vi "Add Dependent File Property.vi"(6 "Node Type":string, 9 "Existing Property Names":string[](array[string]), 10 "Property Parent":string, 11 "Doc Ref":refnum<k20>) -> (1 "Cancelled?":bool, 3 "Property Name out":string, 4 "Node Found?":bool, 5 "Updated Node Ref":refnum<k20>)   [LabVIEW 2025]
panel:
  in  "RT Destination":string
  in  "SupportedTarget":string(combo)="All" caption="Supported Target"
  in  "Version":string
  in  "FIle Path":string
  in  "FileType":string(combo)="To Application Data Dir" caption="File Type"
  in  "ForceDownload":string(combo)="false" caption="Force Download"
  in  "Cancel Button":bool
  in  "Ok Button":bool
  in  "Documentation":string
  in  "Name":string
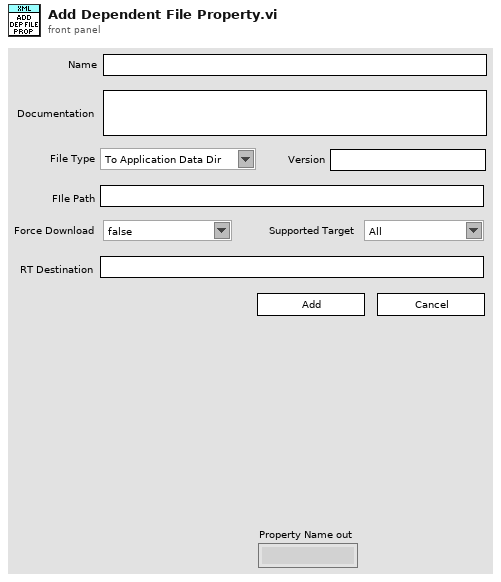
[diagram p1: front panel]
types:
  T1 = cluster{"Name":string, "Documentation":string, "FileType":string, "Version":string, "FIle Path":string, "ForceDownload":string, "SupportedTarget":string, "RT Destination":string}
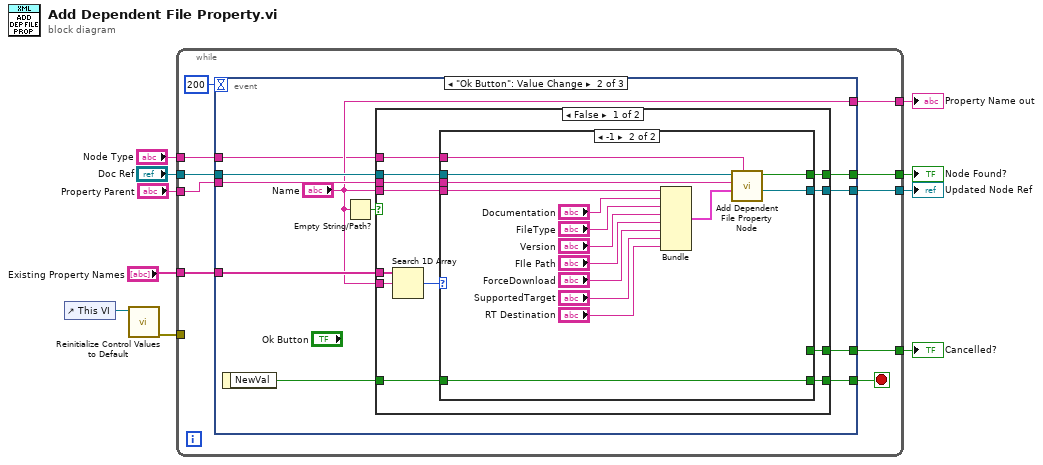
[diagram p0: block diagram]
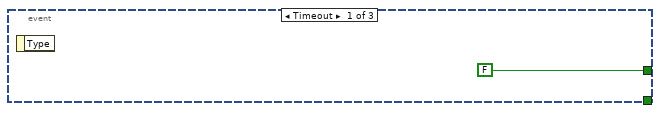
[diagram p2: hidden frame]
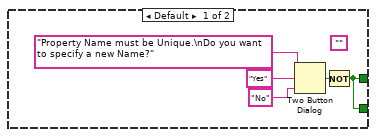
[diagram p3: hidden frame]
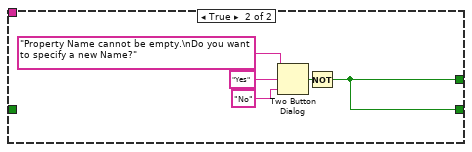
[diagram p4: hidden frame]
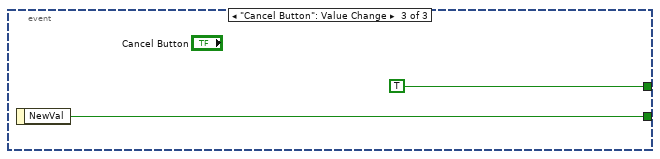
[diagram p5: hidden frame]
diagram:
  n1 = control-ref of="This VI"() -> (w9:refnum<vi>)
  n2 = call "Reinitialize Control Values to Default.vi"("VI Ref"=w9) -> ("error out"=w2:errorcluster)  [unwired: 10 in]
  n3 = while {
    tunnel: "Doc Ref" -> [w20]
    tunnel: [w18] -> w10
    tunnel: "Existing Property Names" -> [w16]
    tunnel: "Property Parent" -> [w15]
    tunnel: [w14] -> w6
    tunnel: [w13] -> w5
    tunnel: "Node Type" -> [w12]
    tunnel: w2 -> [_]
    tunnel: [w11] -> w1
    stop <- w17 stop-if-true
    n4 = event shown="[1] \"Ok Button\": Value Change" {
      selector: _ -> [_ _ _]
      dyn-events: _ -> [_ _ _]
      timeout: 200 -> [_ _ _]
      tunnel: [_ w28 w71] -> w17
      tunnel: w20 -> [_ w31 _]
      tunnel: [FALSE w30 TRUE] -> w18
      tunnel: w16 -> [_ w27 _]
      tunnel: w15 -> [_ w26 _]
      tunnel: [_ "Name" _] -> w14
      tunnel: [_ w24 _] -> w13
      tunnel: w12 -> [_ w23 _]
      tunnel: [_ w22 _] -> w11
      event Timeout {
        n5 = event-data() -> ()  [unwired: 1 in, 1 out]
      }
      event "Ok Button": Value Change {
        n6 = event-data() -> ("NewVal"=w29:bool)  [unwired: 1 in]
        n7 = Empty String/Path?(string/path="Name") -> (empty?=w32:bool)
        n8 = case shown="False" w32 {
          tunnel: w31 -> [w44 _]
          tunnel: "Name" -> [w38 _]
          tunnel: [w43 w65] -> w30
          tunnel: "Name" -> [w42 _]
          tunnel: w29 -> [w41 _]
          tunnel: [w40 w65] -> w28
          tunnel: w27 -> [w39 _]
          tunnel: w26 -> [w36 _]
          tunnel: [w35 _] -> w24
          tunnel: w23 -> [w34 _]
          tunnel: [w33 _] -> w22
          frame False {
            n9 = Search 1D Array(1D array=w39, element=w38) -> (index of element=w37:i32)  [unwired: 1 in]
            n10 = case shown="-1" w37 {
              tunnel: w44 -> [_ w63]
              tunnel: [w45 _] -> w43
              tunnel: w42 -> [_ w59]
              tunnel: [w45 w64] -> w40
              tunnel: w41 -> [_ w64]
              tunnel: w36 -> [_ w62]
              tunnel: [_ w61] -> w35
              tunnel: w34 -> [_ w60]
              tunnel: [_ w50] -> w33
              frame Default {
                (unwired) ""
                n11 = Two Button Dialog(message="Property Name must be Unique.\nDo you want to specify a new Name?" ("Errors"), 1:"No" ("F button name (\"Cancel\")"), 2:"Yes" ("T button name (\"OK\")")) -> (T button?=w46:bool)
                n12 = Not(x=w46) -> (.not. x?=w45:bool)
              }
              frame -1 {
                n13 = Bundle("Name"=w59, "Documentation"="Documentation", "FileType"="FileType", "Version"="Version", "FIle Path"="FIle Path", "ForceDownload"="ForceDownload", "SupportedTarget"="SupportedTarget", "RT Destination"="RT Destination") -> (w51:T1)  [unwired: 1 in]
                n14 = call "Add Dependent File Property Node.vi"("Node Type"=w60, "Dependent File Inputs"=w51, "Property Parent"=w62, "Doc Ref"=w63) -> ("Updated Node Ref"=w50:refnum<k20>, "Node Found?"=w61:bool)  [unwired: 6 in]
              }
            }
          }
          frame True {
            (unwired) ""
            n15 = Two Button Dialog(message="Property Name cannot be empty.\nDo you want to specify a new Name?" ("Errors"), 1:"No" ("F button name (\"Cancel\")"), 2:"Yes" ("T button name (\"OK\")")) -> (T button?=w67:bool)
            n16 = Not(x=w67) -> (.not. x?=w65:bool)
          }
        }
      }
      event "Cancel Button": Value Change {
        n17 = event-data() -> ("NewVal"=w71:bool)  [unwired: 1 in]
      }
    }
  }
  "Cancelled?" <- w10
  "Property Name out" <- w6
  "Node Found?" <- w5
  "Updated Node Ref" <- w1
